vi "Select Two Distinct Cut Indices.vi"(11 "Schedule":u16[](array[numeric])) -> (2 "Index 2":i32, 3 "Index 1":i32)   [LabVIEW 2013, in "GA.lvclass"]
uses:
  GA.lvclass
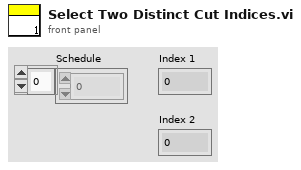
[diagram p1: front panel]
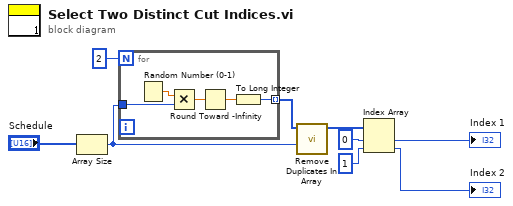
[diagram p0: block diagram]
diagram:
  n1 = Array Size(array="Schedule") -> (size(s)=w5:i32)
  n2 = for {
    N: 2 -> [_]
    tunnel: w5 -> [w11]
    tunnel: [w10] -> w6 mode=indexing
    n3 = Random Number (0-1)() -> (number: 0 to 1=w14:dbl)
    n4 = Multiply(x=w14, y=w11) -> (x*y=w13:dbl)
    n5 = Round Toward -Infinity(1:w13) -> (0:w12:dbl)
    n6 = To Long Integer(number=w12) -> (32bit integer=w10:i32)
  }
  n7 = call "Remove Duplicates In Array.vi"("Max Index Bound"=w5, "Random Numbers Array"=w6) -> ("Random Numbers Array without Duplicates"=w4:i32[])  [unwired: 9 in]
  n8 = Index Array(array=w4, index #1=0 ("index"), index #2=1 ("index")) -> (element #1=→"Index 1":i32, element #2=→"Index 2":i32)
